vi "Queued Query with Result.vi"(6 "result columns (comma list)":string, 8 "error in (no error)":errorcluster, 11 "Query Parameter Data":T2={"UserName"="", "Search Parameters"=[], "eSearch Type"=enum."eSearchFile", "Query Name (vbs)"="Spartan_Query.VBS", "Response queue name"="", "Logic String"=""}) -> (0 "error out":errorcluster, 3 "Query Return Data":T1)   [LabVIEW 2011]
uses:
  DD/lib/Query Result.ctl
  eSearch Types.ctl
  DataFinder Comparisons.ctl
  Datafinder Query.ctl
  DD/lib/Query Queue.ctl
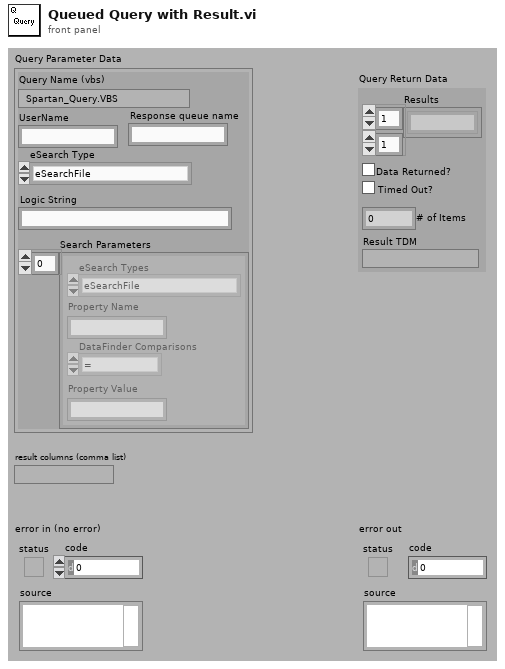
[diagram p1: front panel]
types:
  T1 = typedef "Query Result.ctl" = cluster{"Results":string[][], "# of Items":i32, "Data Returned?":bool, "Result TDM":path, "Timed Out?":bool}
  T2 = typedef "Query Queue.ctl" = cluster{"UserName":string, "Search Parameters":T3[], "eSearch Type":T4, "Query Name (vbs)":string, "Response queue name":string, "Logic String":string}
  T3 = typedef "Datafinder Query.ctl" = cluster{"eSearch Types":T4, "Property Name":string, "DataFinder Comparisons":T5, "Property Value":string}
  T4 = typedef "eSearch Types.ctl" = enum16{"eSearchFile", "eSearchChannelGroup", "eSearchChannel"}
  T5 = typedef "DataFinder Comparisons.ctl" = enum16{"=", "<>", "<", "<=", ">", ">="}
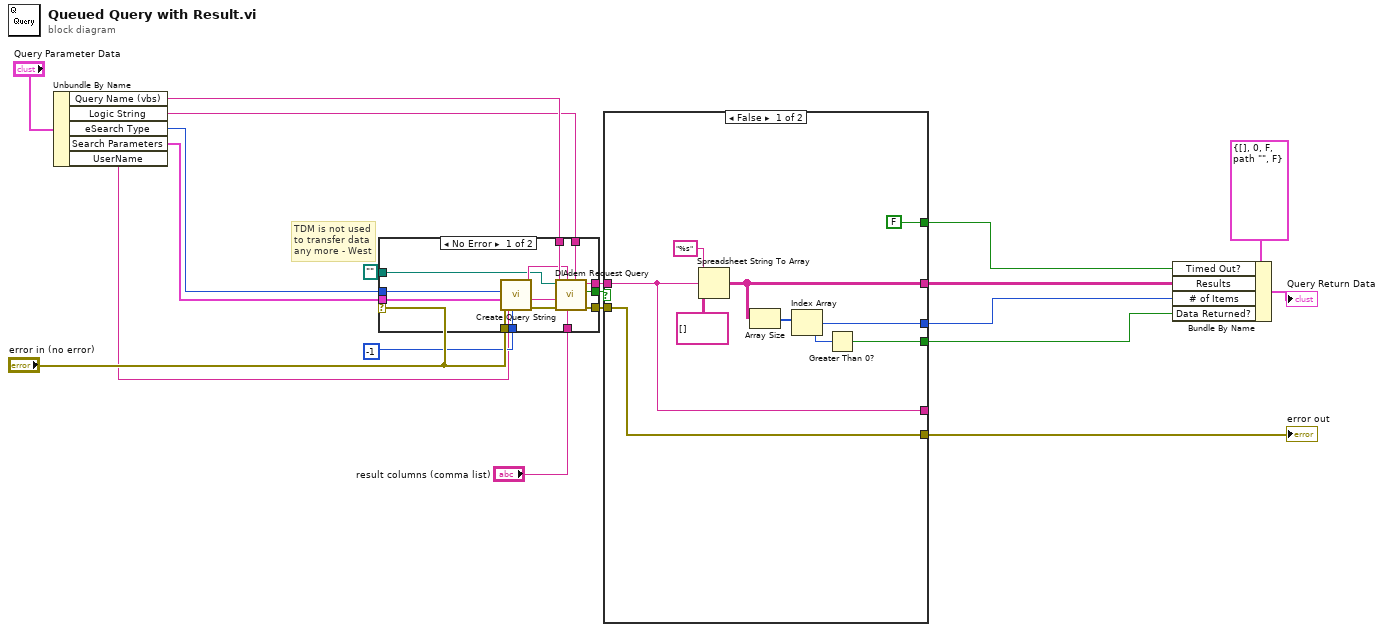
[diagram p0: block diagram]
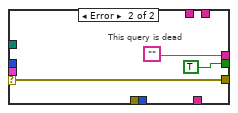
[diagram p2: hidden frame]
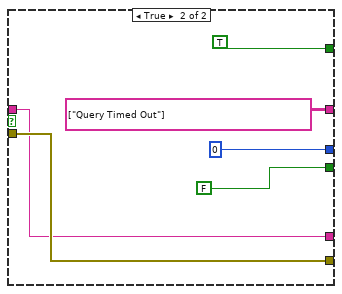
[diagram p3: hidden frame]
diagram:
  # "TDM is not used\nto transfer data\nany more - West"
  n1 = Unbundle By Name("Query Parameter Data") -> ("Query Name (vbs)"=w14:string, "Logic String"=w2:string, "eSearch Type"=w13:T4, "Search Parameters"=w12:T3[], "UserName"=w11:string)
  n2 = case shown="No Error" "error in (no error)" {
    selector: "error in (no error)" -> [_ w37]
    tunnel: [w34 w37] -> w18
    tunnel: w11 -> [w32 _]
    tunnel: w12 -> [w31 _]
    tunnel: w13 -> [w30 _]
    tunnel: [w29 ""] -> w19
    tunnel: path "" -> [w23 _]
    tunnel: -1 ("Max Results (-1 is 5000)") -> [w28 _]
    tunnel: [w27 TRUE ("Timed Out?")] -> w20
    tunnel: w14 -> [w26 _]
    tunnel: "error in (no error)" -> [w25 _]
    tunnel: w2 -> [w22 _]
    tunnel: "result columns (comma list)" -> [w21 _]
    frame No Error {
      n3 = call "Create Query String.vi"("Max Results (-1 is ALL)"=w28, "error in (no error)"=w25, "DataFinder parameters"=w31, "Return Type (ChannelGroup)"=w30) -> ("error out"=w33:errorcluster, "Query String Out"=w24:string)  [unwired: 1 in, 5 out]
      n4 = call "DIAdem Request Query.vi"("Logic String"=w22, "result columns (comma list)"=w21, "Conditions String"=w24, "error in (no error)"=w33, "Username (empty)"=w32, "Query Name"=w26, "Query TDM"=w23) -> ("error out"=w34:errorcluster, "Timed Out?"=w27:bool, "Result"=w29:string)  [unwired: 2 out]
    }
    frame Error {
      # "This query is dead"
    }
  }
  n5 = case shown="False" w20 {
    tunnel: w18 -> [w39 w48]
    tunnel: [w40 string[][] [["Query Timed Out"]] ("Results")] -> w8
    tunnel: [w45 0] -> w5
    tunnel: [w44 FALSE] -> w7
    tunnel: [w39 w48] -> w4
    tunnel: w19 -> [w42 w47]
    tunnel: [FALSE TRUE] -> w9
    tunnel: [w42 w47] -> _
    frame False {
      n6 = Spreadsheet String To Array(format string="%s", spreadsheet string=w42, array type (2D Dbl)=string[][] [] ("Results")) -> (array=w40:string[][])  [unwired: 1 out]
      n7 = Array Size(array=w40) -> (size(s)=w46:i32[])
      n8 = Index Array(array=w46) -> (element=w45:i32)  [unwired: 1 in]
      n9 = Greater Than 0?(x=w45) -> (x > 0?=w44:bool)
    }
    frame True {
    }
  }
  "error out" <- w4
  n10 = Bundle By Name(cluster=T1 {"Results"=[], "# of Items"=0, "Data Returned?"=FALSE, "Result TDM"=path "", "Timed Out?"=FALSE} ("Query Return Data"), "Timed Out?"=w9, "Results"=w8, "# of Items"=w5, "Data Returned?"=w7) -> (→"Query Return Data":T1)
